vi "DARPA_FPGA_DoubleJ_20220715.vi"() -> ()   [LabVIEW 2021]
uses:
  <vilib>/rvi/Emulation/niFpgaGetClockAttributes.vi
  <vilib>/rvi/Emulation/niFpgaSctlEmulationGetInTimedLoop.vi
  <vilib>/rvi/Emulation/niFpgaEmulationReportErrorSimple.vi
  <vilib>/rvi/eio/common/nirviEmuTemplateMethod_errors.vi
  <vilib>/rvi/Emulation/niFpgaProcessEmulError.vi
  <vilib>/rvi/Emulation/niFpgaCriticalErrorInLSC.vi
  <vilib>/eio/EIONode/EIONode.xnode
  <vilib>/rvi/Analysis/measure/butterworth/XNode/niFpgaButterworthFilter.xnode
panel:
  out "t0":u64
  out "Sorted droplet counter":u64=5
  out "t1 (sample)":u64
  out "t0 (sample)":u64
  out "PMT1 sum":u64
  out "PMT2 sum":u64
  out "t1":u64
  out "Droplet counter":u64=53065
  in  "FPGA initializer":bool
  out "loop counter":u64=1
  out "Filtered Signal1":i16
  out "Unfiltered  Signal1":i16
  out "Filtered Signal2":i16
  out "Unfiltered  Signal2":i16
  in  "Threshold1":u64=5000
  in  "Threshold2":u64=1
  out "Loop length (uSec)":u32
  out "Droplet lock on":bool
  out "Where am I":u64=1
  in  "determine ratio":i64
  in  "Time compensation [clock]":i64=5
  out "sample diff":u64
  out "Sort":bool
  out "waveform sort":i16(graph)
  out "waveform wher am i":u64(graph)
  out "waveform PMT1 sum":u64(graph)
  out "waveform PMT2 sum":u64(graph)
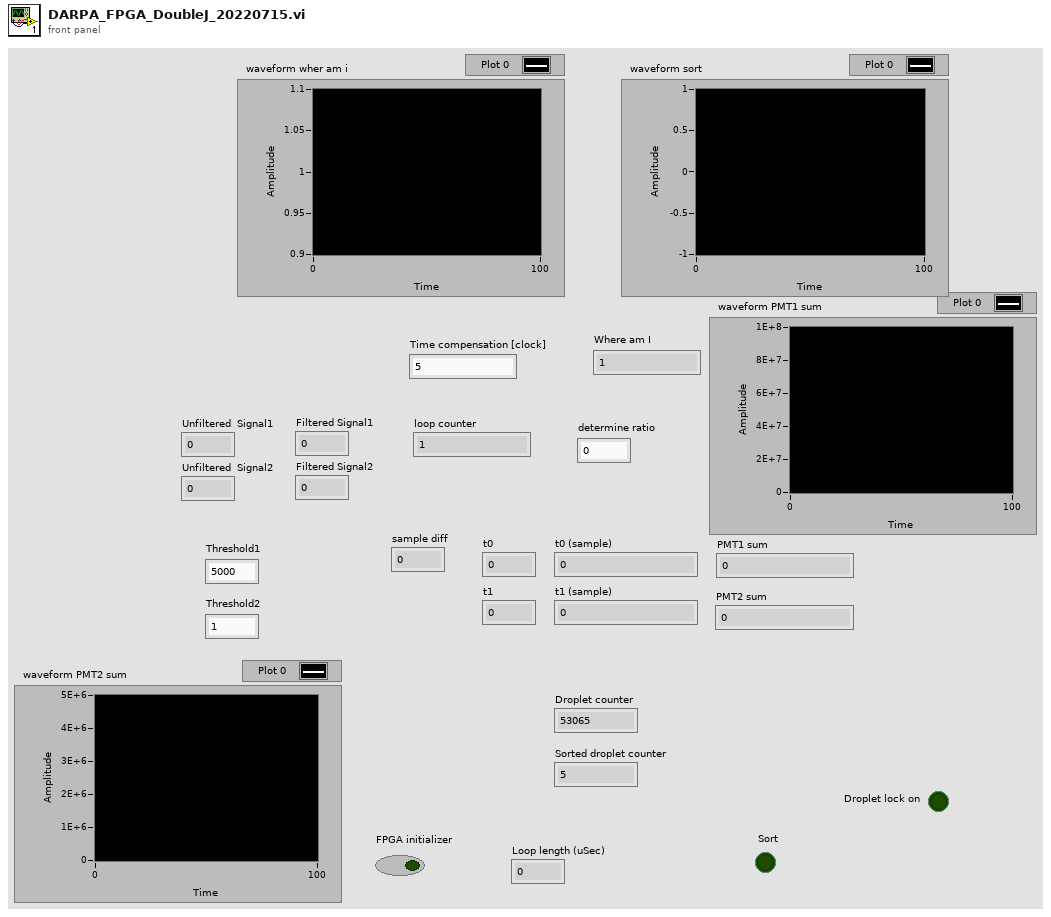
[diagram p1: front panel]
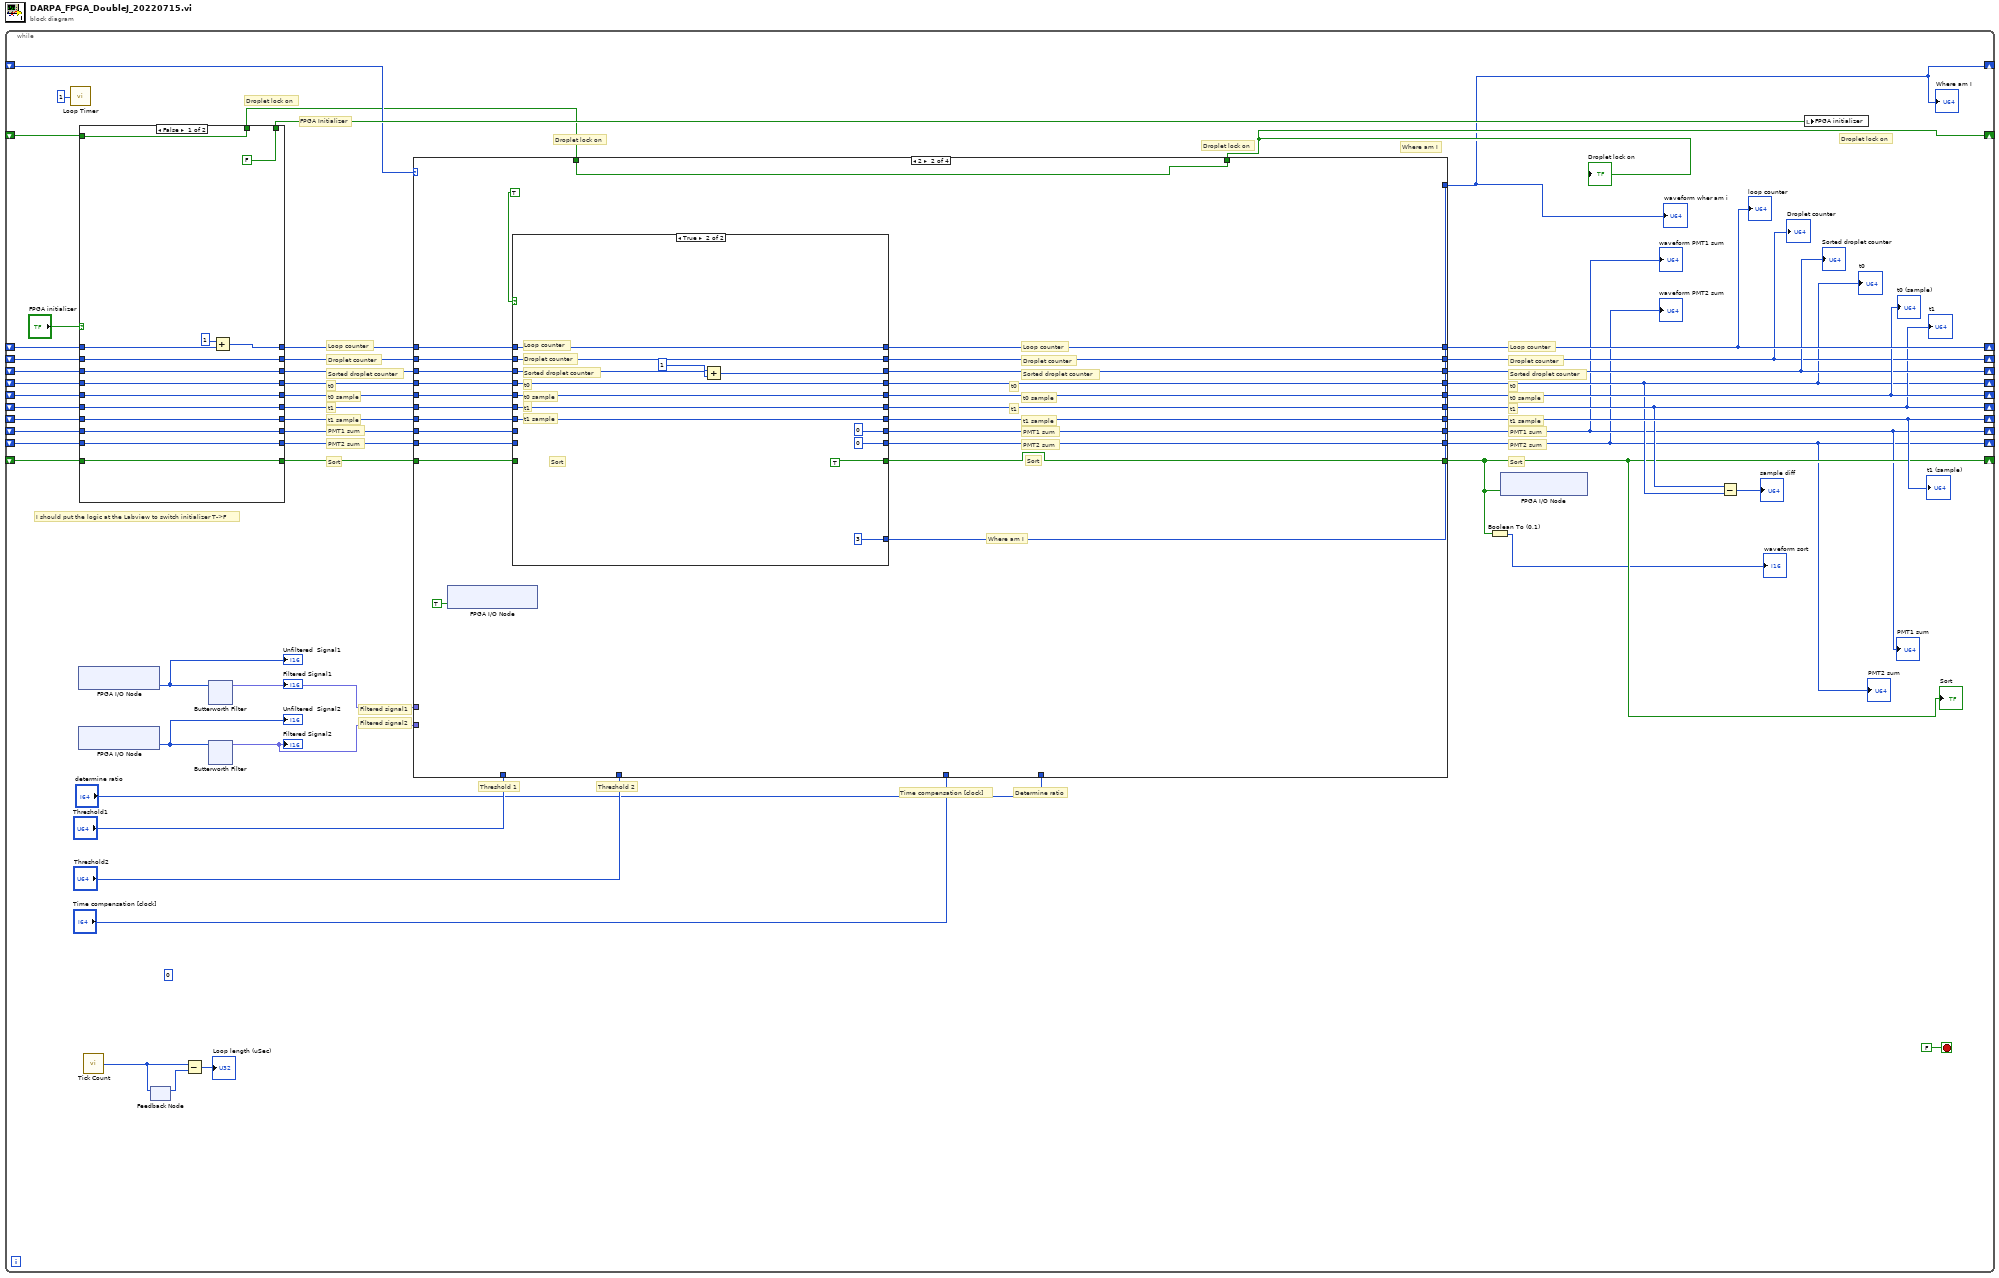
[diagram p0: block diagram]
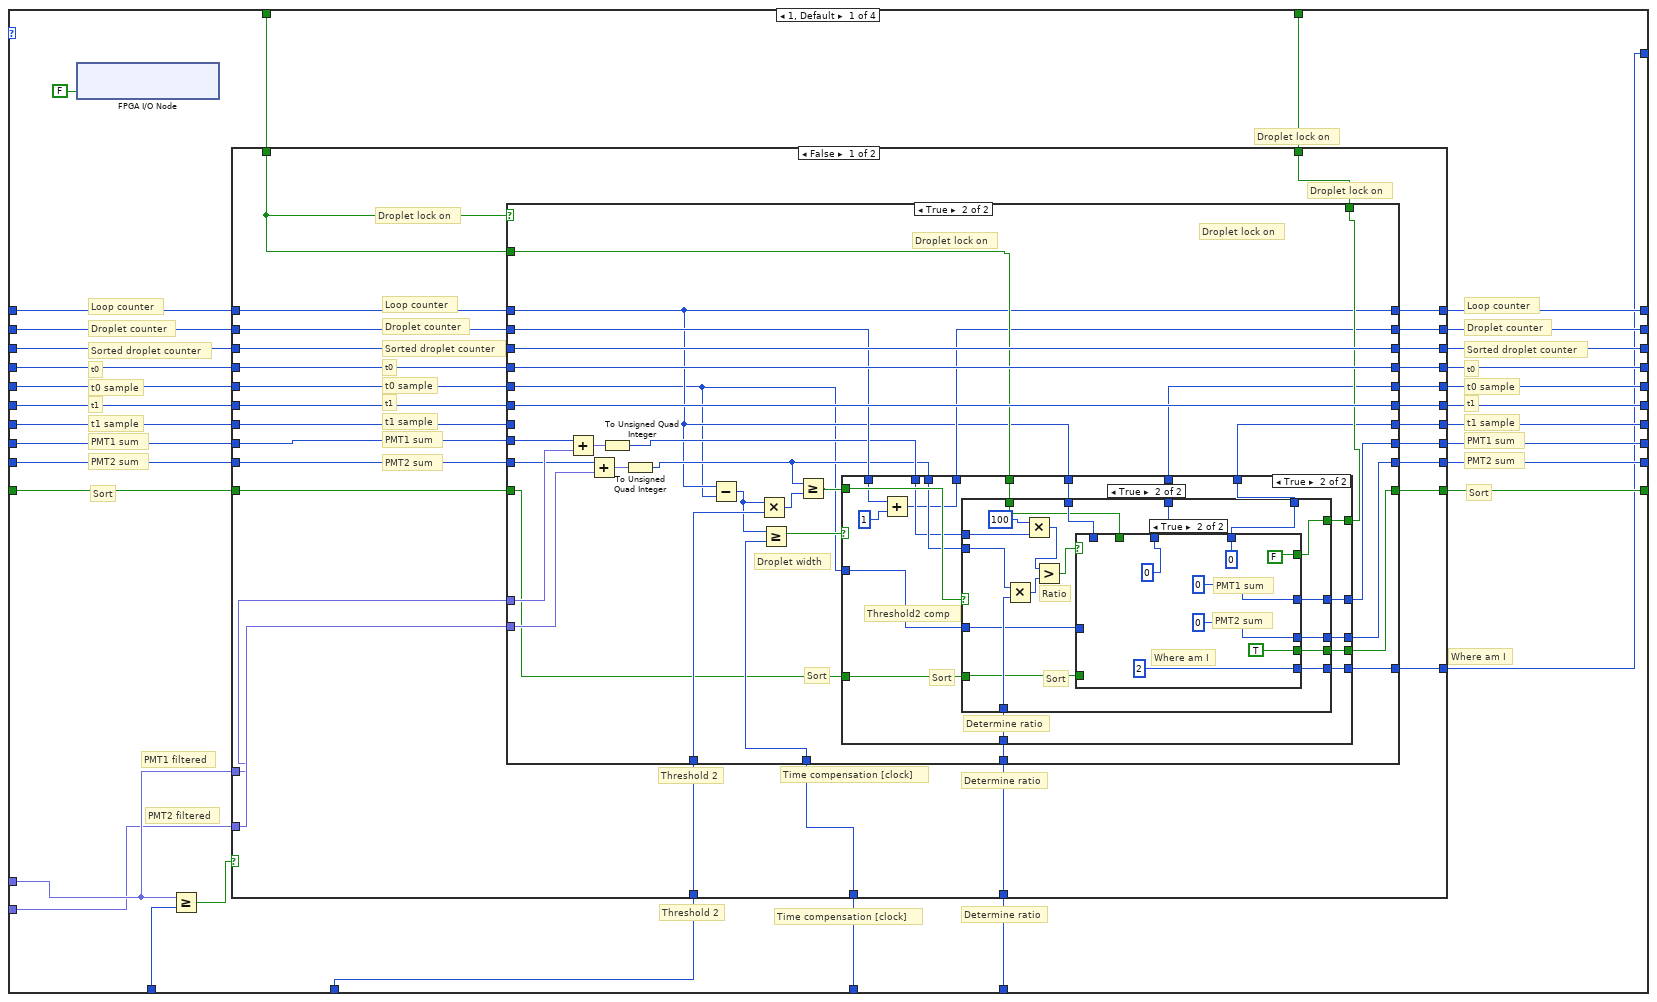
[diagram p2: hidden frame]
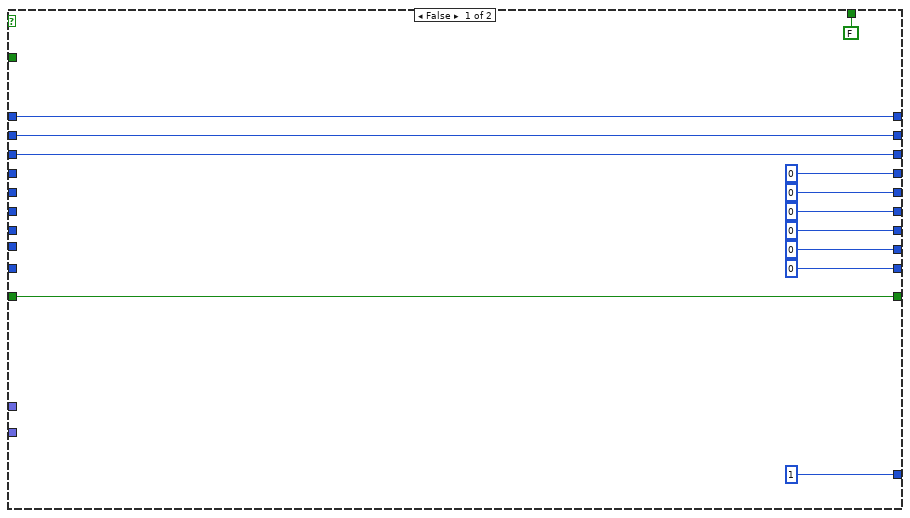
[diagram p3: hidden frame]
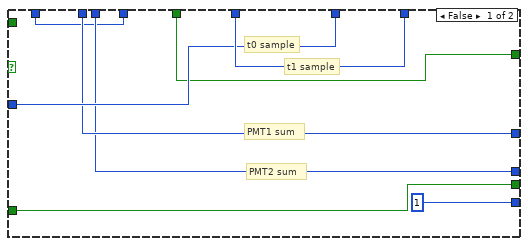
[diagram p4: hidden frame]
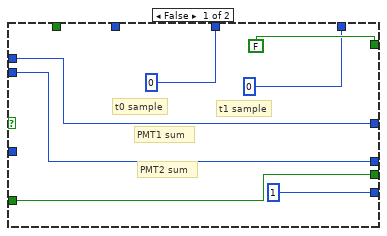
[diagram p5: hidden frame]
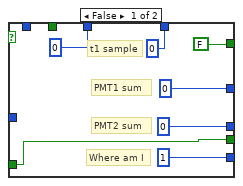
[diagram p6: hidden frame]
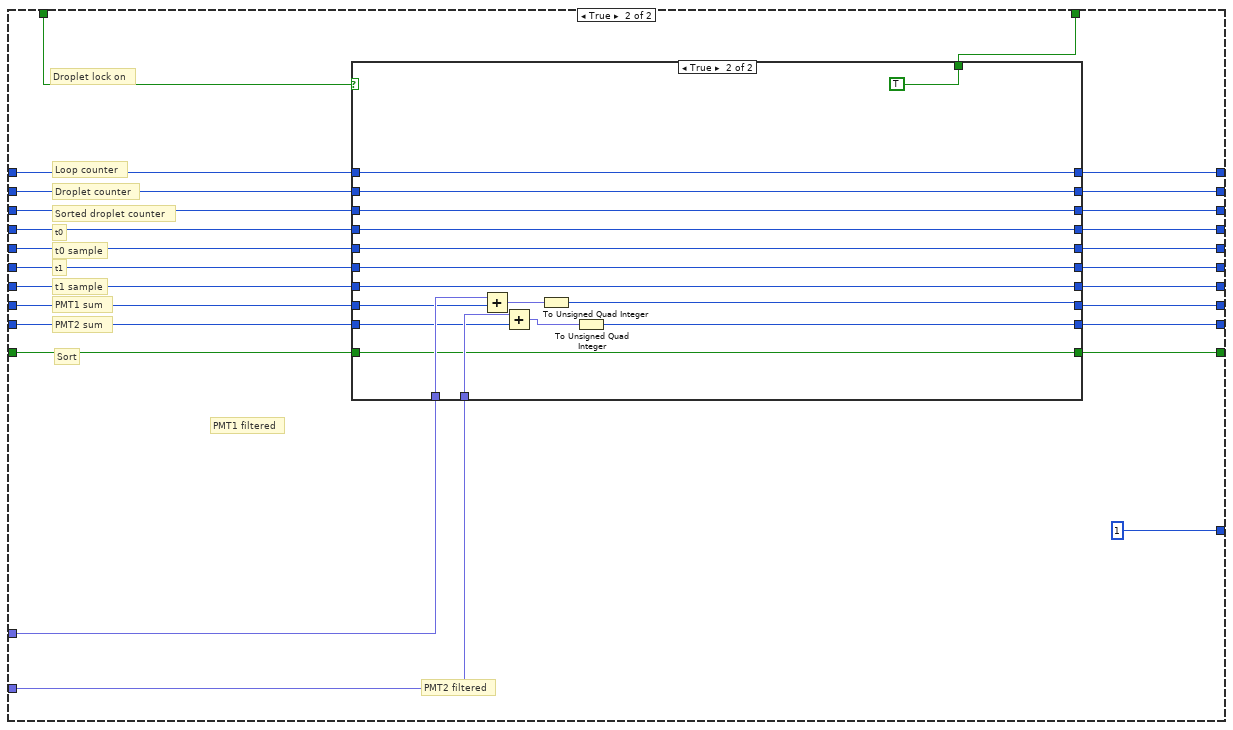
[diagram p7: hidden frame]
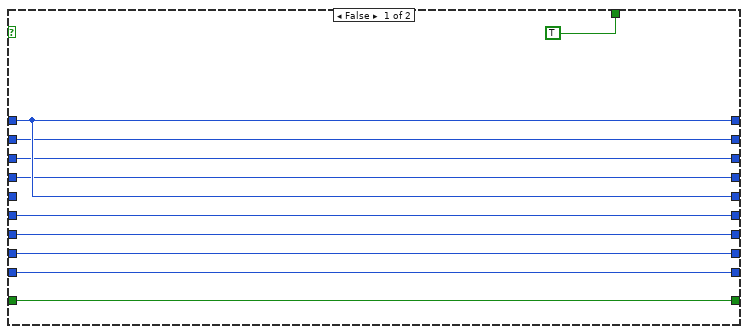
[diagram p8: hidden frame]
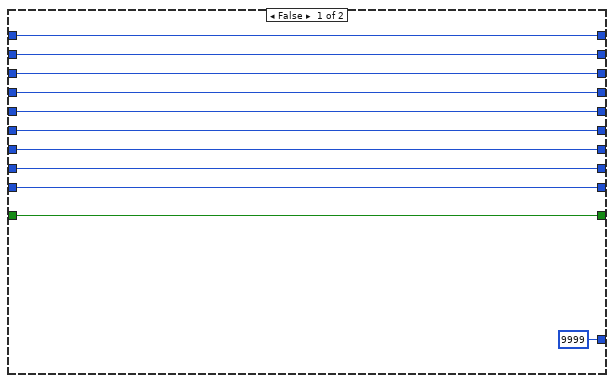
[diagram p9: hidden frame]
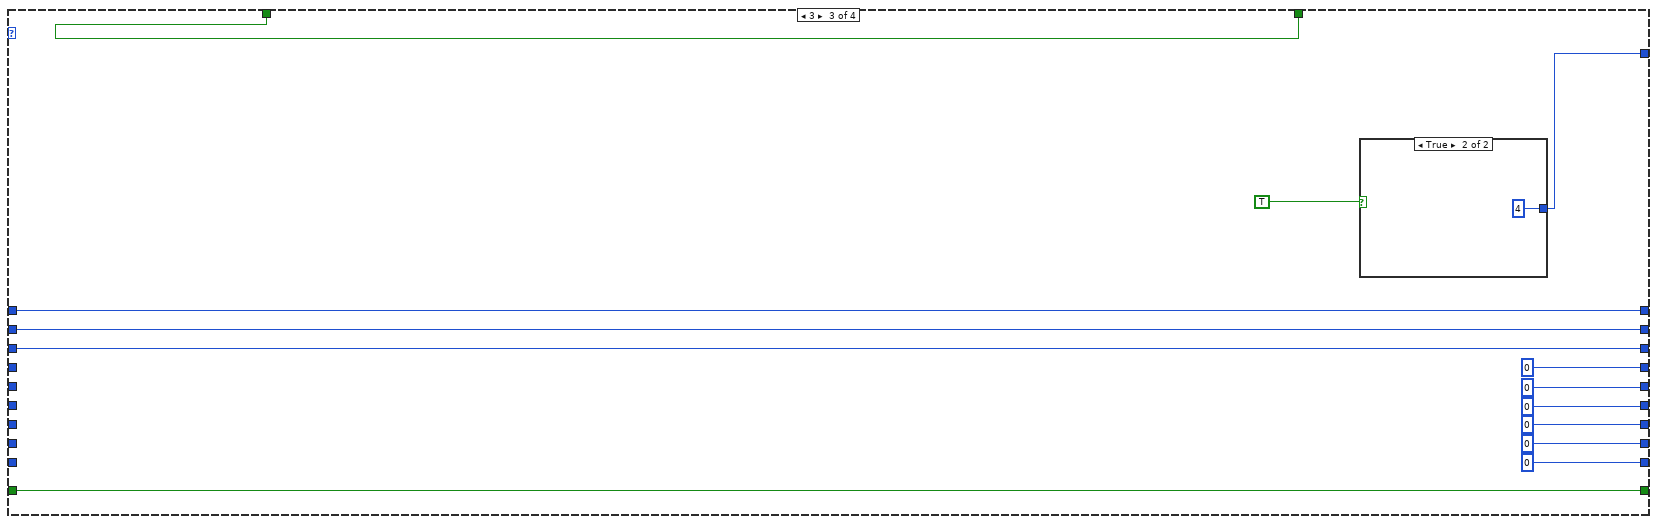
[diagram p10: hidden frame]
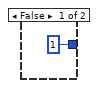
[diagram p11: hidden frame]
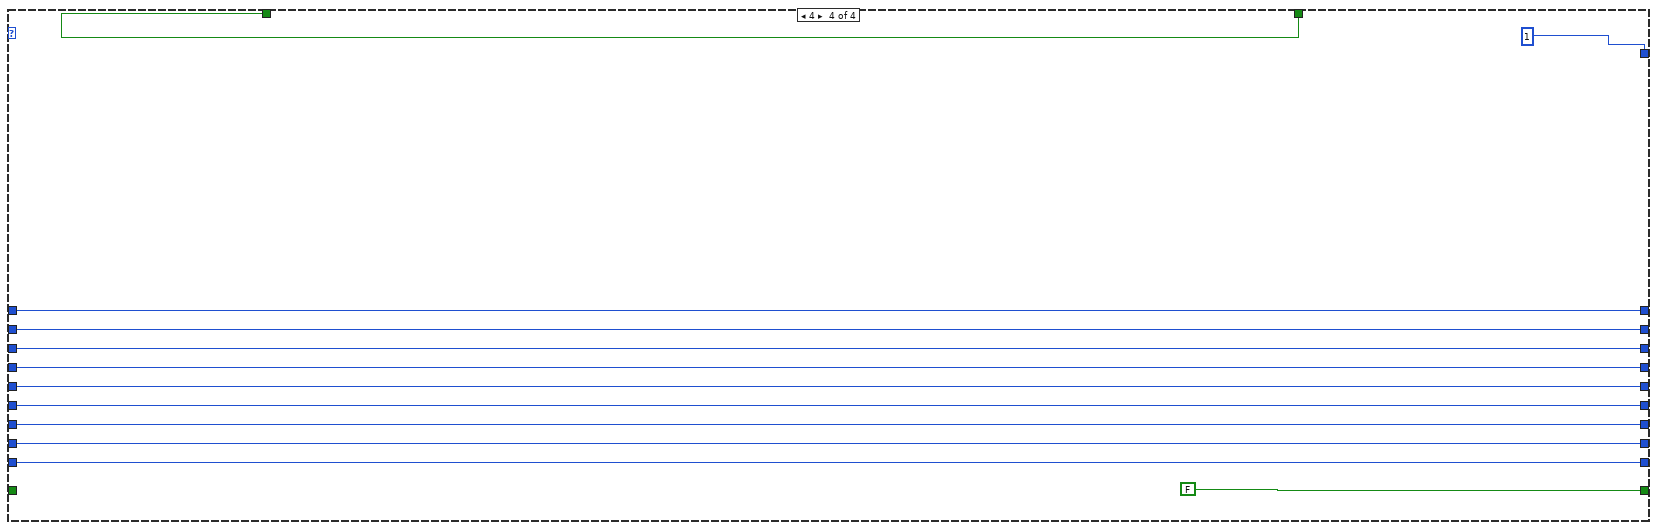
[diagram p12: hidden frame]
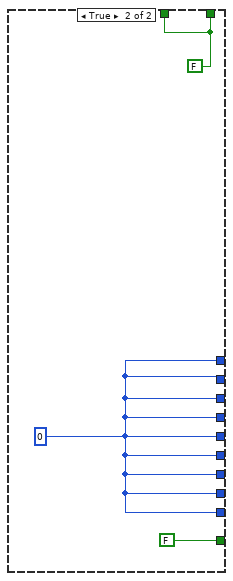
[diagram p13: hidden frame]
diagram:
  n1 = while {
    shift-right: [w28] -> _
    shift-left: _ -> [w50]
    shift-right: [w16] -> _
    shift-left: _ -> [w49]
    shift-right: [w17] -> _
    shift-left: _ -> [w48]
    shift-right: [w7] -> _
    shift-left: _ -> [w47]
    shift-right: [w18] -> _
    shift-left: _ -> [w46]
    shift-right: [w8] -> _
    shift-left: _ -> [w45]
    shift-right: [w19] -> _
    shift-left: _ -> [w44]
    shift-right: [w3] -> _
    shift-left: _ -> [w43]
    shift-right: [w2] -> _
    shift-left: _ -> [w42]
    shift-right: [w32] -> _
    shift-left: _ -> [w36]
    shift-right: [w4] -> _
    shift-left: _ -> [w34]
    shift-right: [w6] -> _
    shift-left: _ -> [w13]
    stop <- FALSE stop-if-true
    (unwired) i16 0
    # "Droplet lock on"
    # "FPGA Initializer"
    # "Where am I"
    # "Droplet lock on"
    # "Time compensation [clock]"
    # "Threshold 2"
    # "Threshold 1"
    # "Determine ratio"
    # "Filtered signal2"
    # "Filtered signal1"
    # "Sort"
    # "PMT2 sum"
    # "PMT1 sum"
    # "t1 sample"
    # "t1"
    # "t0 sample"
    # "t0"
    # "Sorted droplet counter"
    # "Droplet counter"
    # "Loop counter"
    # "Sort"
    # "PMT2 sum"
    # "PMT1 sum"
    # "t1 sample"
    # "t1"
    # "t0 sample"
    # "t0"
    # "Sorted droplet counter"
    # "Droplet counter"
    # "Loop counter"
    # "Droplet lock on"
    # "Droplet lock on"
    # "I should put the logic at the Labview to switch initializer T->F"
    n2 = call "Loop Timer"("Count(Ticks)"=u32 1) -> ()  [unwired: 1 out]
    n3 = xnode "FPGA I/O Node"() -> ("Connector0/AI1"=w41:i16)  [unwired: 1 in, 1 out]
    "Unfiltered  Signal1" <- w41
    n4 = xnode "FPGA I/O Node"() -> ("Connector0/AI2"=w40:i16)  [unwired: 1 in, 1 out]
    "Unfiltered  Signal2" <- w40
    n5 = case shown="False" "FPGA initializer" {
      tunnel: [FALSE ("FPGA initializer") w377] -> w35
      tunnel: [w371 w379] -> w25
      tunnel: [w373 w379] -> w29
      tunnel: [w374 w379] -> w27
      tunnel: [w372 w379] -> w26
      tunnel: [w370 w379] -> w24
      tunnel: [w369 w379] -> w23
      tunnel: [w368 w379] -> w22
      tunnel: [w367 w379] -> w21
      tunnel: [w366 w379] -> w20
      tunnel: w50 -> [w375 _]
      tunnel: w49 -> [w374 _]
      tunnel: w48 -> [w372 _]
      tunnel: w47 -> [w371 _]
      tunnel: w46 -> [w370 _]
      tunnel: w45 -> [w369 _]
      tunnel: w44 -> [w368 _]
      tunnel: w43 -> [w367 _]
      tunnel: w42 -> [w366 _]
      tunnel: [w363 w377] -> w33
      tunnel: w36 -> [w363 _]
      tunnel: w13 -> [w364 _]
      tunnel: [w364 FALSE ("FPGA initializer")] -> w12
      frame False {
        n6 = Add(x=u64 1, y=w375) -> (x+y=w373:u64)
      }
      frame True {
        w379 = u64 0 ("loop counter")
        w377 = FALSE ("FPGA initializer")
      }
    }
    n7 = call "Tick Count"() -> ("Tick Count(uSec)"=w39:u32)
    n8 = feedback #1() -> (w38:u32)  [unwired: 1 in]
    n9 = feedback-in #1(w39) -> ()
    n10 = Subtract(x=w39, y=w38) -> (x-y=→"Loop length (uSec)":u32)
    n11 = xnode "Butterworth Filter"("input data"=w41) -> ("output data"=w15:fxp<+/-,20,20>)  [unwired: 2 in]
    "Filtered Signal1" <- w15
    n12 = xnode "Butterworth Filter"("input data"=w40) -> ("output data"=w14:fxp<+/-,20,20>)  [unwired: 2 in]
    "Filtered Signal2" <- w14
    n13 = case shown="2" w34 {
      tunnel: [w54 w273 w320 i16 1] -> w4
      tunnel: w33 -> [w81 w295 w332 w345]
      tunnel: [w80 w295 w332 w345] -> w32
      tunnel: "Threshold1" -> [w83 _ _ _]
      tunnel: "Threshold2" -> [w57 _ _ _]
      tunnel: w29 -> [w73 w292 w324 w344]
      tunnel: w27 -> [w70 w291 w323 w343]
      tunnel: w26 -> [w69 w290 w322 w342]
      tunnel: w25 -> [w68 w289 _ w341]
      tunnel: w24 -> [w71 w288 _ w340]
      tunnel: w23 -> [w67 w287 _ w339]
      tunnel: w22 -> [w66 w286 _ w338]
      tunnel: w21 -> [w77 w284 _ w337]
      tunnel: w20 -> [w76 w285 _ w336]
      tunnel: [w65 w283 w324 w344] -> w28
      tunnel: [w63 w282 w323 w343] -> w16
      tunnel: [w64 w281 w322 w342] -> w17
      tunnel: [w62 w280 u64 0 ("loop counter") w341] -> w7
      tunnel: [w72 w279 u64 0 ("loop counter") w340] -> w18
      tunnel: [w61 w278 u64 0 ("loop counter") w339] -> w8
      tunnel: [w60 w277 u64 0 ("loop counter") w338] -> w19
      tunnel: [w75 w276 u64 0 ("PMT1 sum") w337] -> w3
      tunnel: [w74 w275 u64 0 ("PMT2 sum") w336] -> w2
      tunnel: w15 -> [w79 _ _ _]
      tunnel: w14 -> [w78 _ _ _]
      tunnel: [w58 w274 w331 FALSE] -> w6
      tunnel: w12 -> [w59 w293 w331 _]
      tunnel: "determine ratio" -> [w55 _ _ _]
      tunnel: "Time compensation [clock]" -> [w56 _ _ _]
      frame 1, Default {
        # "Where am I"
        # "Droplet lock on"
        # "Determine ratio"
        # "Time compensation [clock]"
        # "Threshold 2"
        # "Sort"
        # "PMT2 sum"
        # "PMT1 sum"
        # "t1 sample"
        # "t1"
        # "t0 sample"
        # "t0"
        # "Sorted droplet counter"
        # "Droplet counter"
        # "Loop counter"
        # "Sort"
        # "PMT2 sum"
        # "PMT1 sum"
        # "t1 sample"
        # "t1"
        # "t0 sample"
        # "t0"
        # "Sorted droplet counter"
        # "Droplet counter"
        # "Loop counter"
        # "PMT2 filtered"
        # "PMT1 filtered"
        n14 = xnode "FPGA I/O Node"("Connector0/DIO11"=FALSE) -> ()  [unwired: 1 in, 1 out]
        n15 = Greater Or Equal?(x=w79, y=w83) -> (x >= y?=w82:bool)
        n16 = case shown="False" w82 {
          tunnel: w81 -> [w89 w244]
          tunnel: [w91 w243] -> w80
          tunnel: w79 -> [w84 w240]
          tunnel: w78 -> [w85 w239]
          tunnel: w77 -> [w88 w242]
          tunnel: w76 -> [w87 w241]
          tunnel: [w103 w238] -> w75
          tunnel: [w104 w237] -> w74
          tunnel: w73 -> [w105 w236]
          tunnel: [w100 w235] -> w72
          tunnel: w71 -> [w110 w234]
          tunnel: w70 -> [w106 w233]
          tunnel: w69 -> [w111 w232]
          tunnel: w68 -> [w107 w231]
          tunnel: w67 -> [w108 w230]
          tunnel: w66 -> [w109 w229]
          tunnel: [w96 w228] -> w65
          tunnel: [w98 w227] -> w64
          tunnel: [w97 w226] -> w63
          tunnel: [w99 w225] -> w62
          tunnel: [w101 w224] -> w61
          tunnel: [w102 w223] -> w60
          tunnel: w59 -> [w86 w222]
          tunnel: [w92 w221] -> w58
          tunnel: w57 -> [w95 _]
          tunnel: w56 -> [w94 _]
          tunnel: w55 -> [w93 _]
          tunnel: [w90 u64 1 ("x")] -> w54
          frame False {
            # "Droplet lock on"
            # "Droplet lock on"
            # "Determine ratio"
            # "Time compensation [clock]"
            # "Threshold 2"
            # "PMT2 sum"
            # "PMT1 sum"
            # "t1 sample"
            # "t1"
            # "t0 sample"
            # "t0"
            # "Sorted droplet counter"
            # "Droplet counter"
            # "Loop counter"
            n17 = case shown="True" w89 {
              tunnel: w88 -> [_ w130]
              tunnel: w87 -> [_ w129]
              tunnel: w111 -> [w119 w152]
              tunnel: w110 -> [_ w126]
              tunnel: w109 -> [_ _]
              tunnel: w108 -> [_ w154]
              tunnel: w107 -> [_ w153]
              tunnel: w106 -> [w120 w136]
              tunnel: w105 -> [w115 w127]
              tunnel: [u64 0 ("x") w143] -> w104
              tunnel: [u64 0 ("x") w144] -> w103
              tunnel: [u64 0 ("loop counter") w141] -> w102
              tunnel: [u64 0 ("loop counter") w154] -> w101
              tunnel: [u64 0 ("x") w140] -> w100
              tunnel: [u64 0 ("loop counter") w153] -> w99
              tunnel: [w119 w152] -> w98
              tunnel: [w120 w137] -> w97
              tunnel: [w115 w127] -> w96
              tunnel: w95 -> [_ w151]
              tunnel: w94 -> [_ w138]
              tunnel: w93 -> [_ w146]
              tunnel: w86 -> [w112 w124]
              tunnel: [w112 w125] -> w92
              tunnel: [FALSE ("FPGA initializer") w145] -> w91
              tunnel: [u64 1 ("x") w142] -> w90
              tunnel: w89 -> [_ w139]
              tunnel: w85 -> [_ w133]
              tunnel: w84 -> [_ w132]
              frame False {
              }
              frame True {
                # "Sort"
                # "Droplet width"
                # "Droplet lock on"
                # "Droplet lock on"
                n18 = Add(x=w130, y=w132) -> (x+y=w135:fxp<+/-,64,66>)
                n19 = Add(x=w129, y=w133) -> (x+y=w134:fxp<+/-,64,66>)
                n20 = To Unsigned Quad Integer(1:w135) -> (0:w131:u64)
                n21 = To Unsigned Quad Integer(1:w134) -> (0:w128:u64)
                n22 = Subtract(x=w127, y=w126) -> (x-y=w149:u64)
                n23 = Multiply(x=w149, y=w151) -> (x*y=w150:u64)
                n24 = Greater Or Equal?(x=w149, y=w138) -> (x >= y?=w148:bool)
                n25 = Greater Or Equal?(x=w128, y=w150) -> (x >= y?=w147:bool)
                n26 = case shown="True" w148 {
                  tunnel: w147 -> [_ w180]
                  tunnel: w128 -> [w158 w179]
                  tunnel: w131 -> [w159 w178]
                  tunnel: w146 -> [_ w177]
                  tunnel: [w157 w176] -> w145
                  tunnel: [w159 w175] -> w144
                  tunnel: [w158 w174] -> w143
                  tunnel: [u64 1 ("x") w173] -> w142
                  tunnel: [w161 w172] -> w141
                  tunnel: w127 -> [w161 w171]
                  tunnel: w126 -> [w160 w170]
                  tunnel: [w160 w169] -> w140
                  tunnel: w139 -> [w157 w168]
                  tunnel: w136 -> [w156 w167]
                  tunnel: [w156 w165] -> w137
                  tunnel: [w155 w164] -> w125
                  tunnel: w124 -> [w155 w163]
                  frame False {
                    # "PMT2 sum"
                    # "PMT1 sum"
                    # "t0 sample"
                    # "t1 sample"
                  }
                  frame True {
                    # "Sort"
                    # "Threshold2 comp"
                    # "Determine ratio"
                    n27 = Add(x=w167, y=u64 1) -> (x+y=w165:u64)
                    n28 = case shown="True" w180 {
                      tunnel: w179 -> [w183 w203]
                      tunnel: w178 -> [w182 w192]
                      tunnel: w177 -> [_ w204]
                      tunnel: [FALSE w196] -> w176
                      tunnel: [w182 w201] -> w175
                      tunnel: [w183 w200] -> w174
                      tunnel: [u64 1 ("x") w199] -> w173
                      tunnel: [u64 0 ("loop counter") w198] -> w172
                      tunnel: w171 -> [_ w197]
                      tunnel: w170 -> [_ w194]
                      tunnel: [u64 0 ("loop counter") w193] -> w169
                      tunnel: w168 -> [_ w195]
                      tunnel: [w181 w189] -> w164
                      tunnel: w163 -> [w181 w188]
                      frame False {
                        # "PMT2 sum"
                        # "PMT1 sum"
                        # "t1 sample"
                        # "t0 sample"
                      }
                      frame True {
                        # "Sort"
                        # "Ratio"
                        n29 = Multiply(x=w203, y=w204) -> (x*y=w205:u64)
                        n30 = Multiply(x=u64 100, y=w192) -> (x*y=w190:u64)
                        n31 = Greater?(x=w190, y=w205) -> (0:w202:bool)
                        n32 = case shown="True" w202 {
                          tunnel: [u64 0 ("x") u64 0 ("x")] -> w201
                          tunnel: [u64 0 ("x") u64 0 ("x")] -> w200
                          tunnel: [u64 1 ("x") u64 2 ("x")] -> w199
                          tunnel: [u64 0 ("x") u64 0 ("x")] -> w198
                          tunnel: w197 -> [_ _]
                          tunnel: [FALSE FALSE] -> w196
                          tunnel: w195 -> [_ _]
                          tunnel: w194 -> [_ _]
                          tunnel: [u64 0 ("x") u64 0 ("x")] -> w193
                          tunnel: [w206 TRUE] -> w189
                          tunnel: w188 -> [w206 _]
                          frame False {
                            # "t1 sample"
                            # "Where am I"
                            # "PMT2 sum"
                            # "PMT1 sum"
                          }
                          frame True {
                            # "PMT2 sum"
                            # "PMT1 sum"
                            # "Where am I"
                          }
                        }
                      }
                    }
                  }
                }
              }
            }
          }
          frame True {
            # "Sort"
            # "PMT2 sum"
            # "PMT1 sum"
            # "t1 sample"
            # "t1"
            # "t0 sample"
            # "t0"
            # "Sorted droplet counter"
            # "Droplet counter"
            # "Loop counter"
            # "PMT2 filtered"
            # "PMT1 filtered"
            # "Droplet lock on"
            n33 = case shown="True" w244 {
              tunnel: [TRUE TRUE] -> w243
              tunnel: w242 -> [w253 w270]
              tunnel: w241 -> [w252 w257]
              tunnel: w240 -> [_ w271]
              tunnel: w239 -> [_ w258]
              tunnel: [w253 w268] -> w238
              tunnel: [w252 w266] -> w237
              tunnel: w236 -> [w251 w264]
              tunnel: [w251 w265] -> w235
              tunnel: w234 -> [_ w265]
              tunnel: w233 -> [w249 w263]
              tunnel: w232 -> [w250 w262]
              tunnel: w231 -> [w248 w261]
              tunnel: w230 -> [w247 w260]
              tunnel: w229 -> [w246 w259]
              tunnel: [w251 w264] -> w228
              tunnel: [w250 w262] -> w227
              tunnel: [w249 w263] -> w226
              tunnel: [w248 w261] -> w225
              tunnel: [w247 w260] -> w224
              tunnel: [w246 w259] -> w223
              tunnel: w222 -> [w245 w255]
              tunnel: [w245 w255] -> w221
              frame False {
              }
              frame True {
                n34 = Add(x=w271, y=w270) -> (x+y=w269:fxp<+/-,64,66>)
                n35 = Add(x=w258, y=w257) -> (x+y=w267:fxp<+/-,64,66>)
                n36 = To Unsigned Quad Integer(1:w269) -> (0:w268:u64)
                n37 = To Unsigned Quad Integer(1:w267) -> (0:w266:u64)
              }
            }
          }
        }
      }
      frame 2 {
        # "Sort"
        # "PMT2 sum"
        # "PMT1 sum"
        # "t1 sample"
        # "t1"
        # "t0 sample"
        # "t0"
        # "Sorted droplet counter"
        # "Droplet counter"
        # "Loop counter"
        # "Where am I"
        n38 = xnode "FPGA I/O Node"("Connector0/DIO11"=TRUE) -> ()  [unwired: 1 in, 1 out]
        n39 = case shown="True" TRUE {
          tunnel: w293 -> [w297 _]
          tunnel: w292 -> [w306 w312]
          tunnel: w291 -> [w305 w308]
          tunnel: w290 -> [w304 w311]
          tunnel: w289 -> [w303 w313]
          tunnel: w288 -> [w302 w314]
          tunnel: w287 -> [w301 w315]
          tunnel: w286 -> [w300 w316]
          tunnel: w285 -> [w298 _]
          tunnel: w284 -> [w299 _]
          tunnel: [w306 w312] -> w283
          tunnel: [w305 w308] -> w282
          tunnel: [w304 w309] -> w281
          tunnel: [w303 w313] -> w280
          tunnel: [w302 w314] -> w279
          tunnel: [w301 w315] -> w278
          tunnel: [w300 w316] -> w277
          tunnel: [w299 u64 0 ("PMT1 sum")] -> w276
          tunnel: [w298 u64 0 ("PMT2 sum")] -> w275
          tunnel: [w297 TRUE] -> w274
          tunnel: [u64 9999 ("PMT1 sum") u64 3 ("PMT1 sum")] -> w273
          frame False {
          }
          frame True {
            # "Sort"
            # "t1 sample"
            # "t1"
            # "t0 sample"
            # "t0"
            # "Sorted droplet counter"
            # "Droplet counter"
            # "Loop counter"
            n40 = Add(x=u64 1 ("y"), y=w311) -> (x+y=w309:u64)
          }
        }
      }
      frame 3 {
        n41 = case shown="True" TRUE {
          tunnel: [i16 1 i16 4] -> w320
          frame False {
          }
          frame True {
          }
        }
      }
      frame 4 {
      }
    }
    "t0" <- w7
    "Sorted droplet counter" <- w17
    "t1 (sample)" <- w19
    "t0 (sample)" <- w18
    "PMT1 sum" <- w3
    "PMT2 sum" <- w2
    "t1" <- w8
    "Droplet counter" <- w16
    "loop counter" <- w28
    "Droplet lock on" <- w32
    "Where am I" <- w4
    "Sort" <- w6
    "waveform wher am i" <- w4
    "waveform PMT1 sum" <- w3
    "waveform PMT2 sum" <- w2
    n42 = Boolean To (0,1)(Boolean=w6) -> (0, 1=→"waveform sort":i16)
    n43 = xnode "FPGA I/O Node"("Connector0/DIO1"=w6) -> ()  [unwired: 1 in, 1 out]
    n44 = Subtract(x=w8, y=w7) -> (x-y=→"sample diff":u64)
    n45 = local write "FPGA initializer"(w35) -> ()
  }
